vi "GenerateCode.vi"(1 "Terms":T1[](array[typedef]), 3 "Diagram":refnum<vi>, 5 "XRef":refnum<vi>, 6 "State In":T4) -> (0 "Generated Code?":bool, 2 "State Out":T4, 4 "Reply":string[](array[string]))   [LabVIEW 2018, in "OpenG Remove Duplicates from 1 D Array.xnode"]
uses:
  OpenG Remove Duplicates from 1 D Array.xnode
  State.ctl
  <vilib>/XNodeSupport/XNodeTermIDPair.ctl
  <vilib>/XNodeSupport/XNodeTermRef.ctl
  <vilib>/XNodeSupport/XNodeString.ctl
  <vilib>/Utility/miscctls.llb/LVPositionTypeDef.ctl
  <userlib>/_LAVAcr/Scripting Tools/Scripting Tools.lvlib
  <vilib>/XNodeSupport/NI_XNodeSupport.lvlib
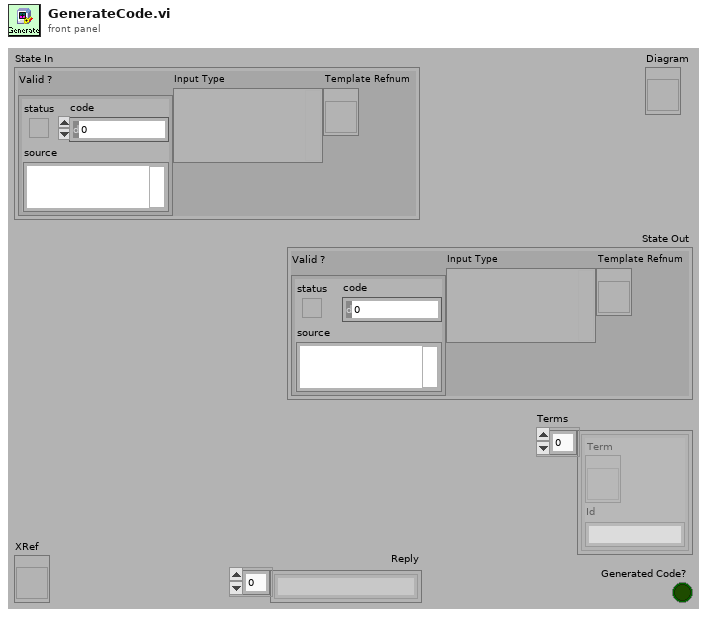
[diagram p1: front panel]
types:
  T1 = typedef "NI_XNodeSupport.lvlib/XNodeTermIDPair.ctl" = cluster{"Term":T2, "Id":T3}
  T2 = typedef "NI_XNodeSupport.lvlib/XNodeTermRef.ctl" = refnum<vi>
  T3 = typedef "NI_XNodeSupport.lvlib/XNodeString.ctl" = string
  T4 = typedef "OpenG Remove Duplicates from 1 D Array.xnode/State.ctl" = cluster{"Valid ?":errorcluster, "Input Type":variant, "Template Refnum":refnum<vi>}
  T5 = typedef "LVPositionTypeDef.ctl" = cluster{"Left":i32, "Top":i32}
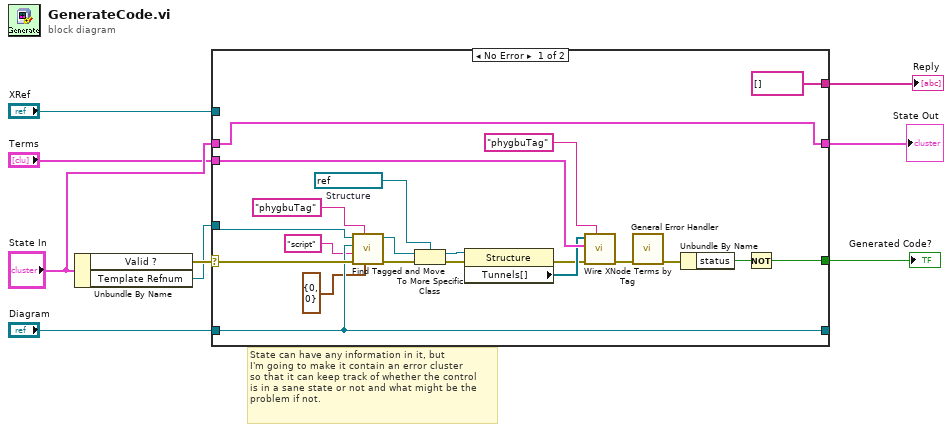
[diagram p0: block diagram]
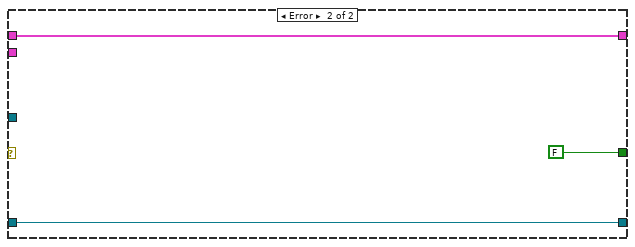
[diagram p2: hidden frame]
diagram:
  # "State can have any information in it, but\nI'm going to make it contain an error cluster\nso that it can keep track of whether the control\nis in a sane state or not and what might be the\nproblem if not."
  n1 = Unbundle By Name("State In") -> ("Valid ?"=w9:errorcluster, "Template Refnum"=w1:refnum<vi>)
  n2 = case shown="No Error" w9 {
    selector: w9 -> [w25 _]
    tunnel: "State In" -> [w29 w33]
    tunnel: "Diagram" -> [w24 w31]
    tunnel: "Terms" -> [w28 _]
    tunnel: "XRef" -> [_ _]
    tunnel: [w24 w31] -> _
    tunnel: [string[] [] ("Reply") _] -> w4
    tunnel: [w17 FALSE] -> w3
    tunnel: [w29 w33] -> w2
    tunnel: w1 -> [w10 _]
    frame No Error {
      w26 = refnum<vi> refnum  # Structure
      n3 = call <userlib>:"Find Tagged and Move.vi"("position"=T5 {"Left"=0, "Top"=0}, "TagName"="phygbuTag", "error in"=w25, "TagValue"="script", "Destination Diagram"=w24, "VI Refnum"=w10) -> ("error out"=w13:errorcluster, "Moved Tagged object"=w15:refnum<vi>)  [unwired: 4 out]
      n4 = To More Specific Class(target class=w26, reference=w15, error in=w13) -> (specific class reference=w27:refnum<vi>, error out=w20:errorcluster)
      n5 = property class="Structure"(reference=w27, error in=w20) -> (error out=w12:errorcluster, "Tunnels[]"=w14:refnum<vi>[])  [unwired: 1 out]
      n6 = call <userlib>:"Wire XNode Terms by Tag.vi"("TagName"="phygbuTag", "error in (no error)"=w12, "Term Refs"=w28, "Source References"=w14) -> ("error out"=w11:errorcluster)  [unwired: 7 out]
      n7 = call <vilib>:"General Error Handler.vi"("error in (no error)"=w11) -> ("error out"=w16:errorcluster)  [unwired: 2 in, 12 out]
      n8 = Unbundle By Name(w16) -> ("status"=w18:bool)
      n9 = Not(x=w18) -> (.not. x?=w17:bool)
    }
    frame Error {
    }
  }
  "State Out" <- w2
  "Reply" <- w4
  "Generated Code?" <- w3
